vi "_PC_Pub getFileExtension.vi"(3 "Input":string) -> (0 "FileName":string, 1 "ExtentionName":string)   [LabVIEW 2018]
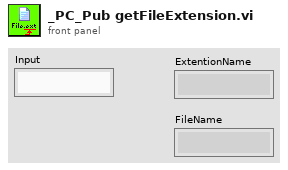
[diagram p1: front panel]
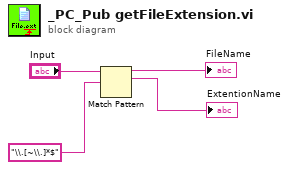
[diagram p0: block diagram]
diagram:
  n1 = Match Pattern(string="Input", regular expression="\\.[~\\.]*$") -> (before substring=→"FileName":string, match substring=→"ExtentionName":string)  [unwired: 1 in, 2 out]
